vi "Test Tree Build.vi"() -> ()   [LabVIEW 2026, in "VILab.lvlib"]
uses:
  VILab.lvlib
  Classes/Tree Manager/Tree Manager.lvclass
  SubVIs/Decompose VI (Refnum).vi
panel:
  out "length":i32
  in  "Tree":string(tree)
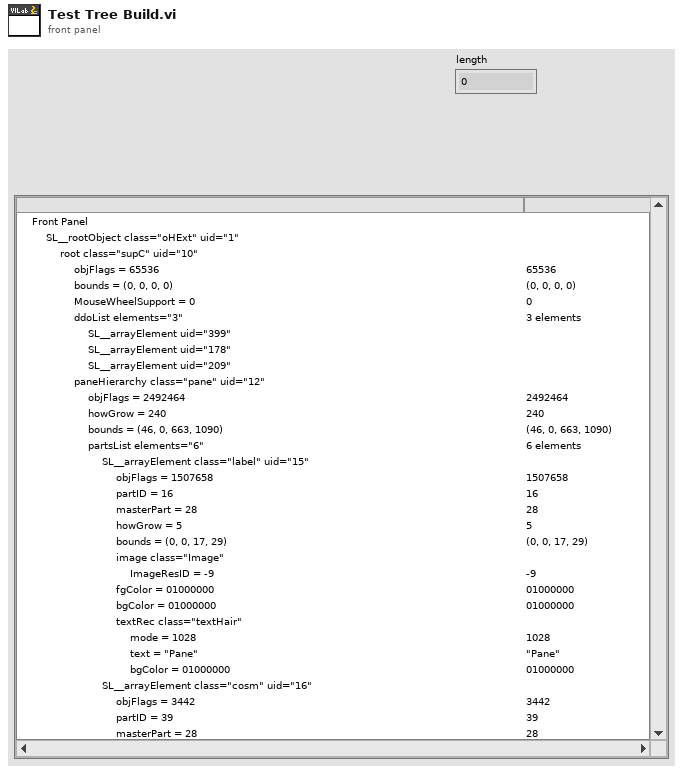
[diagram p1: front panel]
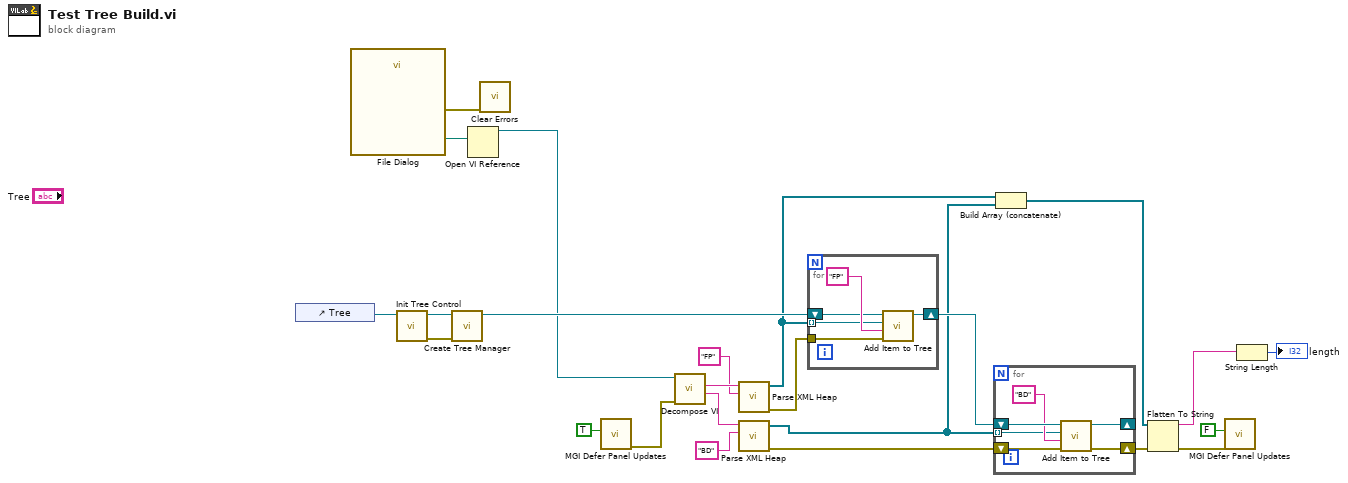
[diagram p0: block diagram]
diagram:
  n1 = control-ref of="Tree"() -> (w17:refnum<vi>)
  n2 = call "File Dialog"() -> ("selected path"=w24:path, "error out"=w23:errorcluster)  [unwired: 12 in, 2 out]
  n3 = call "Init Tree Control.vi"("TreeControl in"=w17) -> ("error out"=w7:errorcluster, "TreeControl out"=w15:refnum<vi>)  [unwired: 9 in]
  n4 = call "Create Tree Manager.vi"("error in (no error)"=w7, "Tree Control"=w15) -> ("Tree Manager"=w16:refnum<class "Tree Manager.lvclass">)  [unwired: 8 in, 1 out]
  n5 = Open VI Reference(vi path=w24) -> (vi reference=w6:refnum<vi>)  [unwired: 5 in, 1 out]
  n6 = call <vilib>:"Clear Errors.vi"("error in (no error)"=w23) -> ()  [unwired: 5 in, 2 out]
  n7 = call <userlib>:"MGI Defer Panel Updates.vi"("Defer Updates?"=TRUE) -> ("Error Out"=w12:errorcluster)  [unwired: 10 in]
  n8 = call-poly "Decompose VI.vi"("error in (no error)"=w12, "VI Ref"=w6) -> ("Block Diagram XML"=w21:string, "Front Panel XML"=w22:string)  [unwired: 5 in, 3 out]
  n9 = call "Parse XML Heap.vi"("Root Parent"="FP" ("Parent Tag"), "XML"=w22) -> ("error out"=w18:errorcluster, "Items"=w3:refnum<class "Data Item.lvclass">[])  [unwired: 8 in]
  n10 = call "Parse XML Heap.vi"("Root Parent"="BD" ("Parent Tag"), "XML"=w21) -> ("error out"=w19:errorcluster, "Items"=w2:refnum<class "Data Item.lvclass">[])  [unwired: 8 in]
  n11 = for {
    tunnel: w18 -> [w28]
    shift-right: [w29] -> w20
    shift-left: w16 -> [w26]
    tunnel: w3 -> [w25] mode=indexing
    n12 = call "Add Item to Tree.vi"("error in (no error)"=w28, "Parent Tag"="FP", "Data Item"=w25, "Tree Manager in"=w26) -> ("Tree Manager out"=w29:refnum<class "Tree Manager.lvclass">)  [unwired: 5 in, 2 out]
  }
  n13 = for {
    shift-right: [w32] -> _
    shift-left: w20 -> [w35]
    shift-right: [w31] -> w11
    shift-left: w19 -> [w34]
    tunnel: w2 -> [w30] mode=indexing
    n14 = call "Add Item to Tree.vi"("error in (no error)"=w34, "Parent Tag"="BD", "Data Item"=w30, "Tree Manager in"=w35) -> ("error out"=w31:errorcluster, "Tree Manager out"=w32:refnum<class "Tree Manager.lvclass">)  [unwired: 5 in, 1 out]
  }
  n15 = Build Array (concatenate)(w3, w2) -> (w1:refnum<class "Data Item.lvclass">[])
  n16 = Flatten To String(anything=w1, error in (no error)=w11) -> (data string=w14:string, error out=w8:errorcluster)  [unwired: 2 in, 1 out]
  n17 = call <userlib>:"MGI Defer Panel Updates.vi"("Error In"=w8, "Defer Updates?"=FALSE) -> ()  [unwired: 9 in, 1 out]
  n18 = String Length(string=w14) -> (length=→"length":i32)
